vi "pcfs_dither_loop.vi"(8 "error in (no error)":errorcluster, 11 "pcfs in":refnum<class "pcfs.lvclass">) -> (0 "error out":errorcluster, 3 "pcfs out":refnum<class "pcfs.lvclass">)   [LabVIEW 2015, in "pcfs.lvclass"]
uses:
  pcfs.lvclass
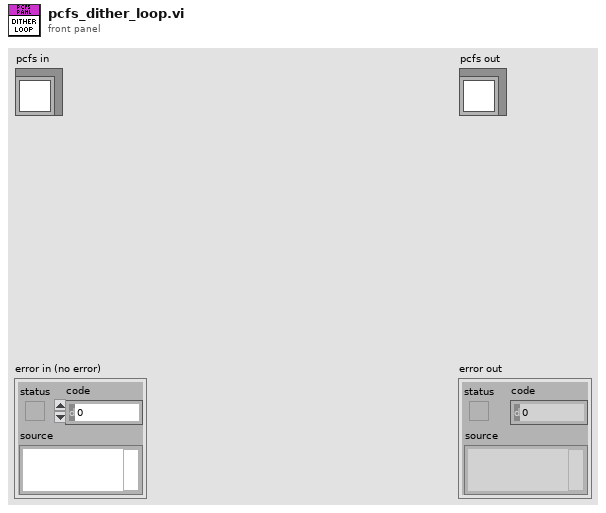
[diagram p1: front panel]
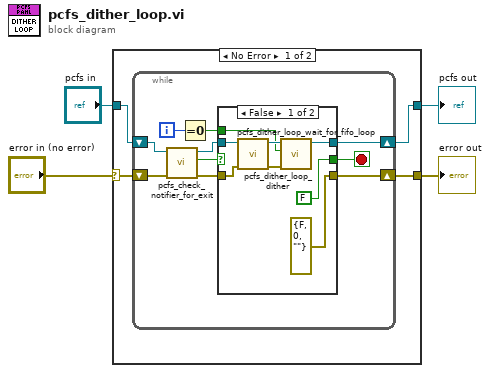
[diagram p0: block diagram]
diagram:
  n1 = case shown="No Error" "error in (no error)" {
    selector: "error in (no error)" -> [w7 w31]
    tunnel: [w6 w31] -> w3
    tunnel: [w5 w30] -> w1
    tunnel: "pcfs in" -> [w8 w30]
    frame No Error {
      n2 = while {
        shift-right: [w12] -> w5
        shift-left: w8 -> [w18]
        shift-right: [w11] -> w6
        shift-left: w7 -> [w17]
        i -> [w10]
        stop <- w15 stop-if-true
        n3 = call "pcfs_check_notifier_for_exit.vi"("error in (no error)"=w17, "pcfs in"=w18) -> ("error out"=w14:errorcluster, "exit?"=w16:bool, "pcfs out"=w13:refnum<class "pcfs.lvclass">)  [unwired: 7 in]
        n4 = Equal To 0?(x=w10) -> (x = 0?=w9:bool)
        n5 = case shown="False" w16 {
          selector: w16 -> [_ w29]
          tunnel: [FALSE w29] -> w15
          tunnel: w14 -> [w26 w27]
          tunnel: w13 -> [w25 w28]
          tunnel: [w21 w28] -> w12
          tunnel: [errorcluster {"status"=FALSE, "code"=0, "source"=""} ("error out") w27] -> w11
          tunnel: w9 -> [w19 _]
          frame False {
            n6 = call "pcfs_dither_loop_wait_for_fifo_loop.vi"("error in (no error)"=w26, "pcfs in"=w25) -> ("error out"=w23:errorcluster, "pcfs out"=w22:refnum<class "pcfs.lvclass">)  [unwired: 8 in]
            n7 = call "pcfs_dither_loop_dither.vi"("error in (no error)"=w23, "first_dither?"=w19, "pcfs in"=w22) -> ("pcfs out"=w21:refnum<class "pcfs.lvclass">)  [unwired: 7 in, 1 out]
          }
          frame True {
          }
        }
      }
    }
    frame Error {
    }
  }
  "error out" <- w3
  "pcfs out" <- w1
